vi "createEvents.vi"(8 "error in (no error)":errorcluster, 11 "SnapperEvents in":refnum<class "SnapperEvents.lvclass">) -> (0 "error out":errorcluster, 3 "SnapperEvents out":refnum<class "SnapperEvents.lvclass">)   [LabVIEW 2009, in "Views.lvlib" / "Camera.lvlib" / "SnapperEvents.lvclass"]
uses:
  SnapperEvents.lvclass
  SnapperEvents.lvclass/SnapperEvents.ctl
  Camera.lvlib
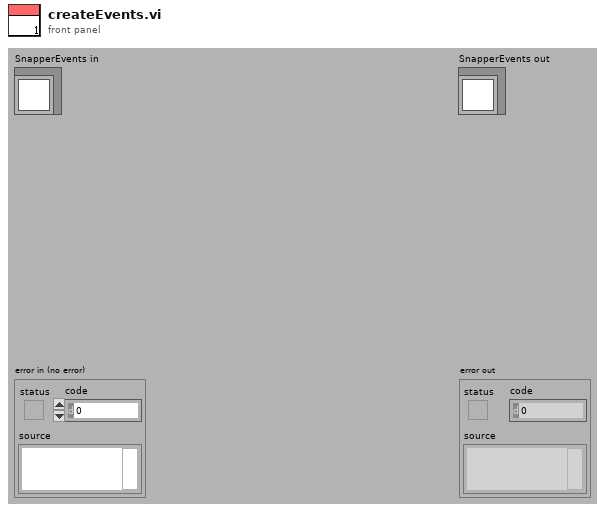
[diagram p1: front panel]
types:
  T1 = cluster{"frontEndEvents":cluster{"snapShotEvent":refnum<user-event>, "stopShooting":refnum<user-event>, "userSnapShot":refnum<user-event>}, "backEndEvents":cluster{"picture":refnum<user-event>}}
  T2 = cluster{"Path":path, "atomNumber":dbl, "xWidth":dbl, "zWidth":dbl}
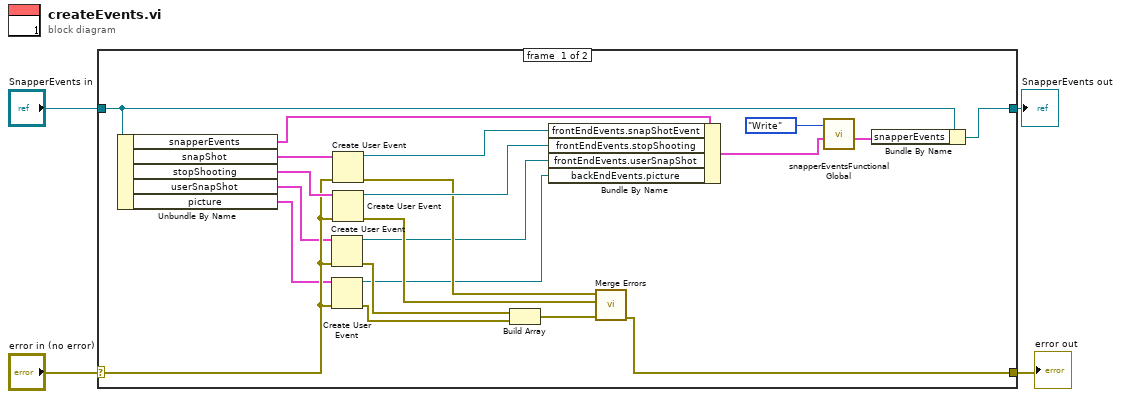
[diagram p0: block diagram]
diagram:
  n1 = case shown="No Error" "error in (no error)" {
    selector: "error in (no error)" -> [w15 w27]
    tunnel: [w22 w27] -> w3
    tunnel: [w25 w26] -> w1
    tunnel: "SnapperEvents in" -> [w24 w26]
    frame #0 {
      n2 = Unbundle By Name(w24) -> ("snapperEvents"=w12:T1, "snapShot"=w21:cluster{"pictureDir":path}, "stopShooting"=w20:cluster{"dummy":bool}, "userSnapShot"=w13:cluster{"pictureDir":path}, "picture"=w14:T2)
      n3 = Create User Event(user event datatype=w13, error in=w15) -> (user event=w11:refnum<user-event>, error out=w10:errorcluster)
      n4 = Create User Event(user event datatype=w14, error in=w15) -> (user event=w5:refnum<user-event>, error out=w9:errorcluster)
      n5 = Create User Event(user event datatype=w21, error in=w15) -> (user event=w19:refnum<user-event>, error out=w17:errorcluster)
      n6 = Create User Event(user event datatype=w20, error in=w15) -> (user event=w18:refnum<user-event>, error out=w16:errorcluster)
      n7 = Build Array(w10, w9) -> (w8:errorcluster[])
      n8 = Bundle By Name(cluster=w12, "frontEndEvents.snapShotEvent"=w19, "frontEndEvents.stopShooting"=w18, "frontEndEvents.userSnapShot"=w11, "backEndEvents.picture"=w5) -> (w6:T1)
      n9 = call <vilib>:"Merge Errors.vi"("error array in"=w8, "error in 2 (no error)"=w16, "error in 1 (no error)"=w17) -> ("error out"=w22:errorcluster)  [unwired: 4 in]
      n10 = call "snapperEventsFunctionalGlobal.vi"("snapperEvents"=w6, "Action"=enum16{"Write", "Read"}."Write") -> ("snapperEvents"=w7:T1)  [unwired: 9 in]
      n11 = Bundle By Name(cluster=w24, "snapperEvents"=w7) -> (w25:refnum<class "SnapperEvents.lvclass">)
    }
    frame #1 {
    }
  }
  "error out" <- w3
  "SnapperEvents out" <- w1
